vi "write to stdout.vi"(10 "data":string) -> ()   [LabVIEW 2024]
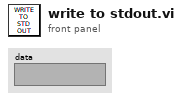
[diagram p1: front panel]
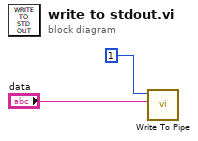
[diagram p0: block diagram]
diagram:
  n1 = call <vilib>:"Write To Pipe.vi"("data"="data", "file descriptor"=1) -> ()  [unwired: 3 in, 3 out]
